vi "ErrorCode.vi"(10 "parent VI path":path, 11 "return type":i32) -> (3 "error out":errorcluster)   [LabVIEW 2023, in "RDB.lvlib"]
uses:
  RDB.lvlib
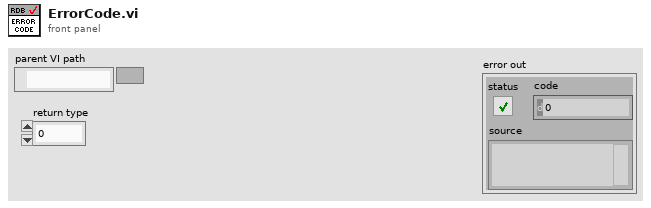
[diagram p1: front panel]
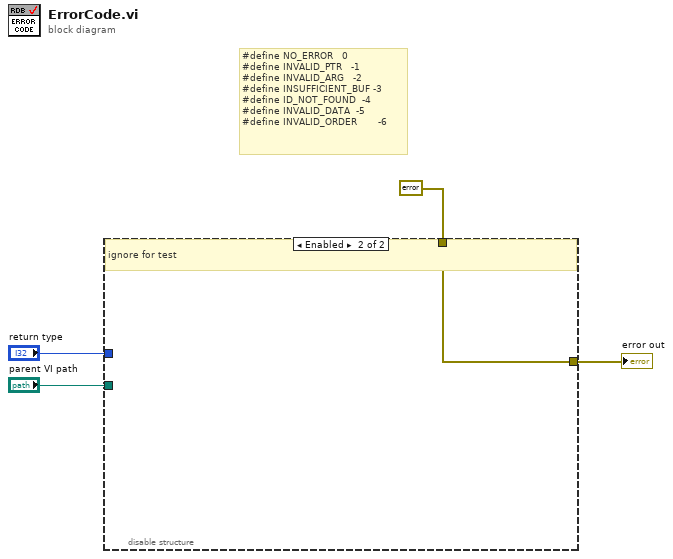
[diagram p0: block diagram]
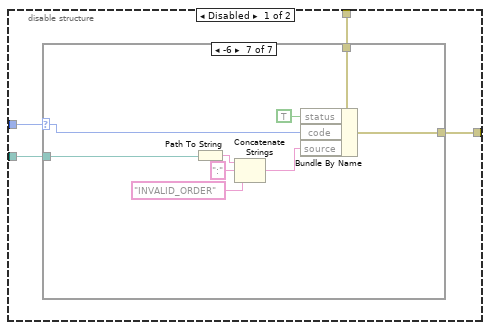
[diagram p2: hidden frame]
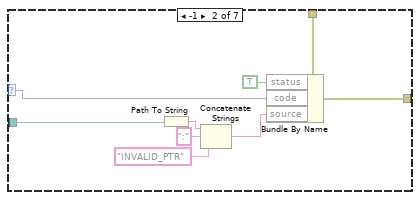
[diagram p4: hidden frame]
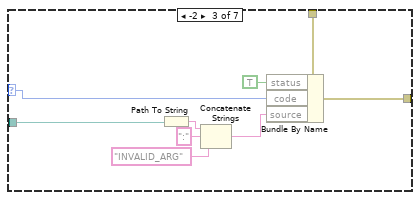
[diagram p5: hidden frame]
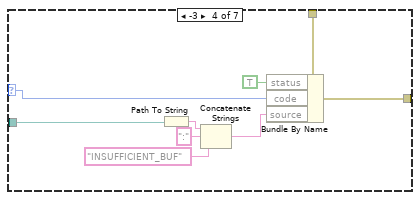
[diagram p6: hidden frame]
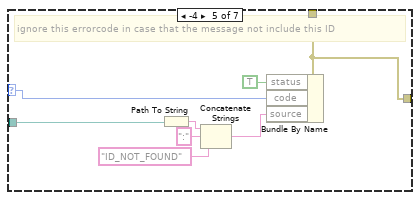
[diagram p7: hidden frame]
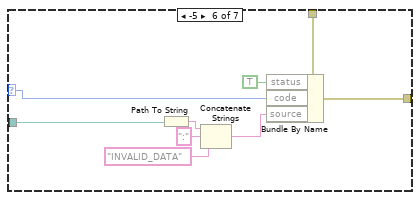
[diagram p8: hidden frame]
diagram:
  # "#define NO_ERROR\t\t\t0\n#define INVALID_PTR\t\t\t-1\n#define INVALID_ARG\t\t\t-2\n#define INSUFFICIENT_BUF\t-3\n#define ID_NOT_FOUND\t\t-4\n#define INVALID_DATA\t\t-5\n#define INVALID_ORDER       -6"
  n1 = disable-structure shown="Enabled" {
    disable-tunnel: "return type" -> [w8 _]
    disable-tunnel: errorcluster {"status"=FALSE, "code"=0, "source"=""} ("error in (no error)") -> [w7 w63]
    disable-tunnel: [w6 w63] -> w2
    disable-tunnel: "parent VI path" -> [w5 _]
    frame Disabled {
      n2 = case shown="-6" w8 {
        selector: w8 -> [_ w17 w26 w35 w44 w52 w61]
        tunnel: w7 -> [w9 w18 w27 w36 w37 w53 w62]
        tunnel: [w9 w11 w20 w29 w37 w46 w55] -> w6
        tunnel: w5 -> [_ w10 w19 w28 w38 w45 w54]
        frame 0, Default {
        }
        frame -1 {
          n3 = Path To String(path=w10) -> (string=w15:string)
          n4 = Concatenate Strings(w15, ":" ("string"), "INVALID_PTR" ("string")) -> (w12:string)
          n5 = Bundle By Name(cluster=w18, "status"=TRUE, "code"=w17, "source"=w12) -> (w11:errorcluster)
        }
        frame -2 {
          n6 = Path To String(path=w19) -> (string=w24:string)
          n7 = Concatenate Strings(w24, ":" ("string"), "INVALID_ARG" ("string")) -> (w21:string)
          n8 = Bundle By Name(cluster=w27, "status"=TRUE, "code"=w26, "source"=w21) -> (w20:errorcluster)
        }
        frame -3 {
          n9 = Path To String(path=w28) -> (string=w33:string)
          n10 = Concatenate Strings(w33, ":" ("string"), "INSUFFICIENT_BUF" ("string")) -> (w30:string)
          n11 = Bundle By Name(cluster=w36, "status"=TRUE, "code"=w35, "source"=w30) -> (w29:errorcluster)
        }
        frame -4 {
          # "ignore this errorcode in case that the message not include this ID"
          n12 = Path To String(path=w38) -> (string=w42:string)
          n13 = Concatenate Strings(w42, ":" ("string"), "ID_NOT_FOUND" ("string")) -> (w39:string)
          n14 = Bundle By Name(cluster=w37, "status"=TRUE, "code"=w44, "source"=w39) -> ()  [unwired: 1 out]
        }
        frame -5 {
          n15 = Path To String(path=w45) -> (string=w50:string)
          n16 = Concatenate Strings(w50, ":" ("string"), "INVALID_DATA" ("string")) -> (w47:string)
          n17 = Bundle By Name(cluster=w53, "status"=TRUE, "code"=w52, "source"=w47) -> (w46:errorcluster)
        }
        frame -6 {
          n18 = Path To String(path=w54) -> (string=w59:string)
          n19 = Concatenate Strings(w59, ":" ("string"), "INVALID_ORDER" ("string")) -> (w56:string)
          n20 = Bundle By Name(cluster=w62, "status"=TRUE, "code"=w61, "source"=w56) -> (w55:errorcluster)
        }
      }
    }
    frame Enabled {
      # "ignore for test"
    }
  }
  "error out" <- w2
